vi "Main.vi"() -> ()   [LabVIEW 2017]
doc: "This Continuous Measurement sample project is based on the Queued Message Handler template.\n\nThe Event Handling Loop generates messages based on user interface actions.\n\nThe Message Handling Loop processes messages generated by the Event Handling Loop, or by other messages. There are also Acquisition and Logging message handling loop subVIs, and a chart updating loop."
uses:
  Acquisition/Hardware Configuration.ctl
  Logging/Logging Configuration.ctl
  <vilib>/Analysis/baseanly.llb/Mean (DBL).vi
  <vilib>/express/express analysis/Spectral/Block/exnSpectralBlock spectral measurements PSD poly.vi
  <vilib>/express/express analysis/Spectral/Block/exnSpectralBlock spectral measurements PSD DDT.vi
  support/Message Queue/Enqueue Message (Single).vi
  <vilib>/Utility/error.llb/Error Cluster From Error Code.vi
  <vilib>/express/express analysis/Spectral/XNode/ExpressSpectralMeasurementsBlockNode.xnode
  <vilib>/ErrorRing/Error Ring.xnode
  Acquisition/Acquisition.lvlib
  Logging/Logging.lvlib
  Settings/Settings.lvlib
  support/User Event - Stop/User Event - Stop.lvlib
  support/Message Queue/Message Queue.lvlib
  <vilib>/Analysis/NI_AALBase.lvlib
  <vilib>/gmath/NI_Gmath.lvlib
panel:
  out "XY Graph 4":cluster{"Y":sgl[], "Y":sgl[]}(graph)
  in  "Plot 2":bool
  out "XY Graph 3":cluster{"Y":sgl[], "Y":sgl[]}(graph)
  out "B2Y 2":dbl(graph)=nan
  out "B2X 3":dbl(graph)=nan
  out "B1Y 2":dbl(graph)=nan
  out "B1X 2":dbl(graph)=nan
  out "B2X 2":dbl(graph)
  out "PZTZ0":dbl
  out "PZTY0":dbl
  out "PZTX0":dbl
  in  "PZTZ_offset":dbl caption="Offset" format="%#.0f"
  in  "PZTY_offset":dbl caption="Offset" format="%#.0f"
  in  "PZTX_offset":dbl caption="Offset" format="%#.0f"
  in  "Plot":bool
  in  "PSD":bool
  in  "PZT_offset":bool caption="Offset all"
  out "PZTZ PSD":dynamicdata(graph)=[{"t0"=timestamp(0 s since 1904-01-01), "dt"=inf, "Y"=[], "attributes"=variant("NI_ChannelName"=variant(string "Collected (PSD)"), "NI_OriginalChannelName"=variant(string "Collected"))}]
  out "PZTY PSD":dynamicdata(graph)=[{"t0"=timestamp(0 s since 1904-01-01), "dt"=inf, "Y"=[], "attributes"=variant("NI_ChannelName"=variant(string "Collected (PSD)"), "NI_OriginalChannelName"=variant(string "Collected"))}]
  out "PZTX PSD":dynamicdata(graph)=[{"t0"=timestamp(0 s since 1904-01-01), "dt"=inf, "Y"=[], "attributes"=variant("NI_ChannelName"=variant(string "Collected (PSD)"), "NI_OriginalChannelName"=variant(string "Collected"))}]
  in  "B1X":dbl=1.0
  in  "B1Y":dbl=1.0
  in  "B2X":dbl=1.0
  in  "B2Y":dbl=1.0
  out "Description":string
  out "User":string
  out "Corr":dbl format="%.2g"
  out "XY Graph 2":cluster{"Y":sgl[], "Y":sgl[]}(graph) caption="XY Graph"
  out "Corr":dbl format="%.2g"
  out "XY Graph":cluster{"Y":sgl[], "Y":sgl[]}(graph)
  out "B2S":sgl format="%#_2g"
  out "B2Y":dbl(graph)=nan
  out "B2X":dbl(graph)=nan
  out "B2Y PSD":dynamicdata(graph)=[{"t0"=timestamp(0 s since 1904-01-01), "dt"=inf, "Y"=[], "attributes"=variant("NI_ChannelName"=variant(string "Collected (PSD)"), "NI_OriginalChannelName"=variant(string "Collected"))}]
  out "B2X PSD":dynamicdata(graph)=[{"t0"=timestamp(0 s since 1904-01-01), "dt"=inf, "Y"=[], "attributes"=variant("NI_ChannelName"=variant(string "Collected (PSD)"), "NI_OriginalChannelName"=variant(string "Collected"))}]
  out "B1S":sgl format="%#_2g"
  out "B1Y PSD":dynamicdata(graph)=[{"t0"=timestamp(0 s since 1904-01-01), "dt"=inf, "Y"=[], "attributes"=variant("NI_ChannelName"=variant(string "Collected (PSD)"), "NI_OriginalChannelName"=variant(string "Collected"))}]
  out "B1X PSD":dynamicdata(graph)=[{"t0"=timestamp(0 s since 1904-01-01), "dt"=inf, "Y"=[], "attributes"=variant("NI_ChannelName"=variant(string "Collected (PSD)"), "NI_OriginalChannelName"=variant(string "Collected"))}]
  out "PZTZ":dbl(graph)
  out "PZTY":dbl(graph)
  out "PZTX":dbl(graph)
  out "?":dbl
  out "Input (V)":dbl
  out "Rate (Hz)":dbl
  in  "Stop_Log":bool
  in  "Log":bool
  in  "Exit":bool
  out "Status":string
  in  "Settings":bool
  in  "Stop_Acquire":bool
  in  "Acquire":bool
  out "B1Y":dbl(graph)=nan
  out "B1X":dbl(graph)=nan
  # "nm/V"
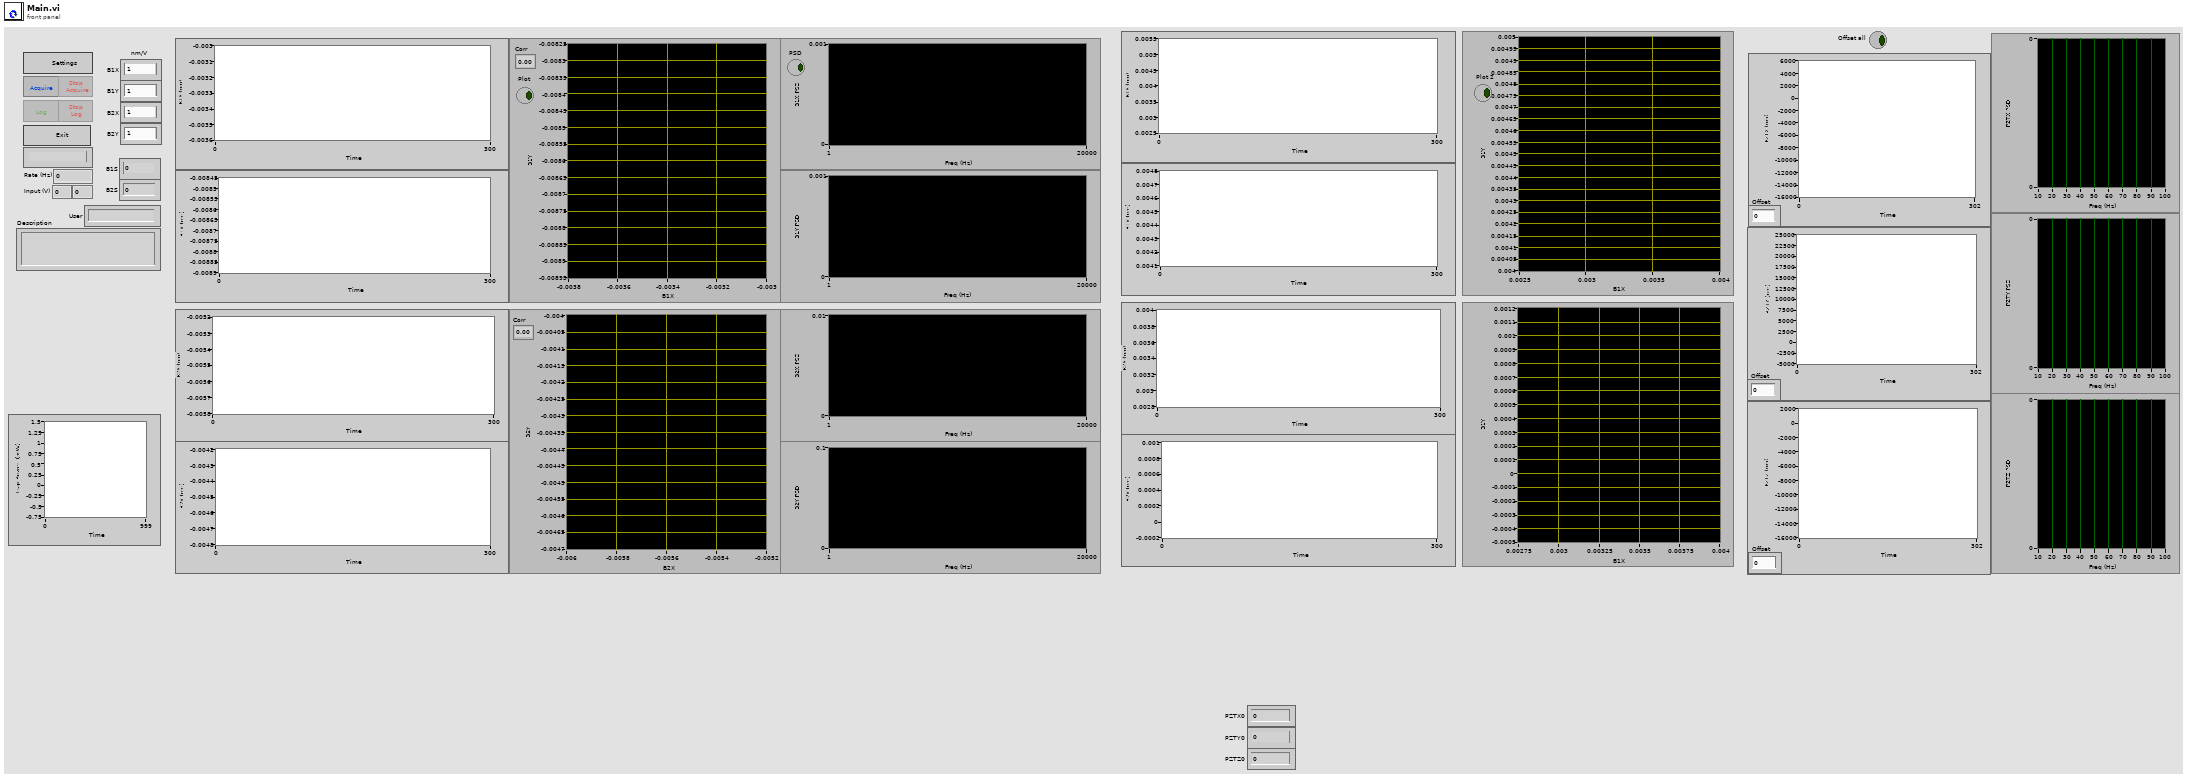
[diagram p1: front panel]
types:
  T1 = cluster{"Acquire Ref":refnum<vi>, "Log Ref":refnum<vi>, "Stop_Acquire Ref":refnum<vi>, "Settings Ref":refnum<vi>, "Status Ref":refnum<vi>, "Exit Ref":refnum<vi>, "Stop_Log Ref":refnum<vi>}
  T2 = typedef "Acquisition.lvlib/Hardware Configuration.ctl" = cluster{"DAQmx Input":tag, "Max Input":dbl, "Min Input":dbl, "Sample Rate":dbl, "DAQmx Task":refnum<k21>}
  T3 = typedef "Logging.lvlib/Logging Configuration.ctl" = cluster{"Log File Base Path":path, "TDMS File Reference":refnum<k34>, "Channel names":string[], "Author":string, "Description":string}
  T4 = cluster{"Hardware Configuration":T2, "Logging Configuration":T3}
  T5 = typedef "Message Queue.lvlib/All Message Queues.ctl" = cluster{"UI":refnum<queue>, "Acquisition":refnum<queue>, "Logging":refnum<queue>}
  T6 = cluster{"averaging mode":u16, "weighting mode":u16, "number of averages":u32}
  T7 = cluster{"dB On (F)":bool, "unwrap phase (F)":bool, "convert to degree (F)":bool}
  T8 = cluster{"Hardware Configuration":T2, "Logging Configuration":cluster{"Log File Base Path":path, "TDMS File Reference":refnum<k34>, "Channel names":string[], "Author":string, "Description":string}}
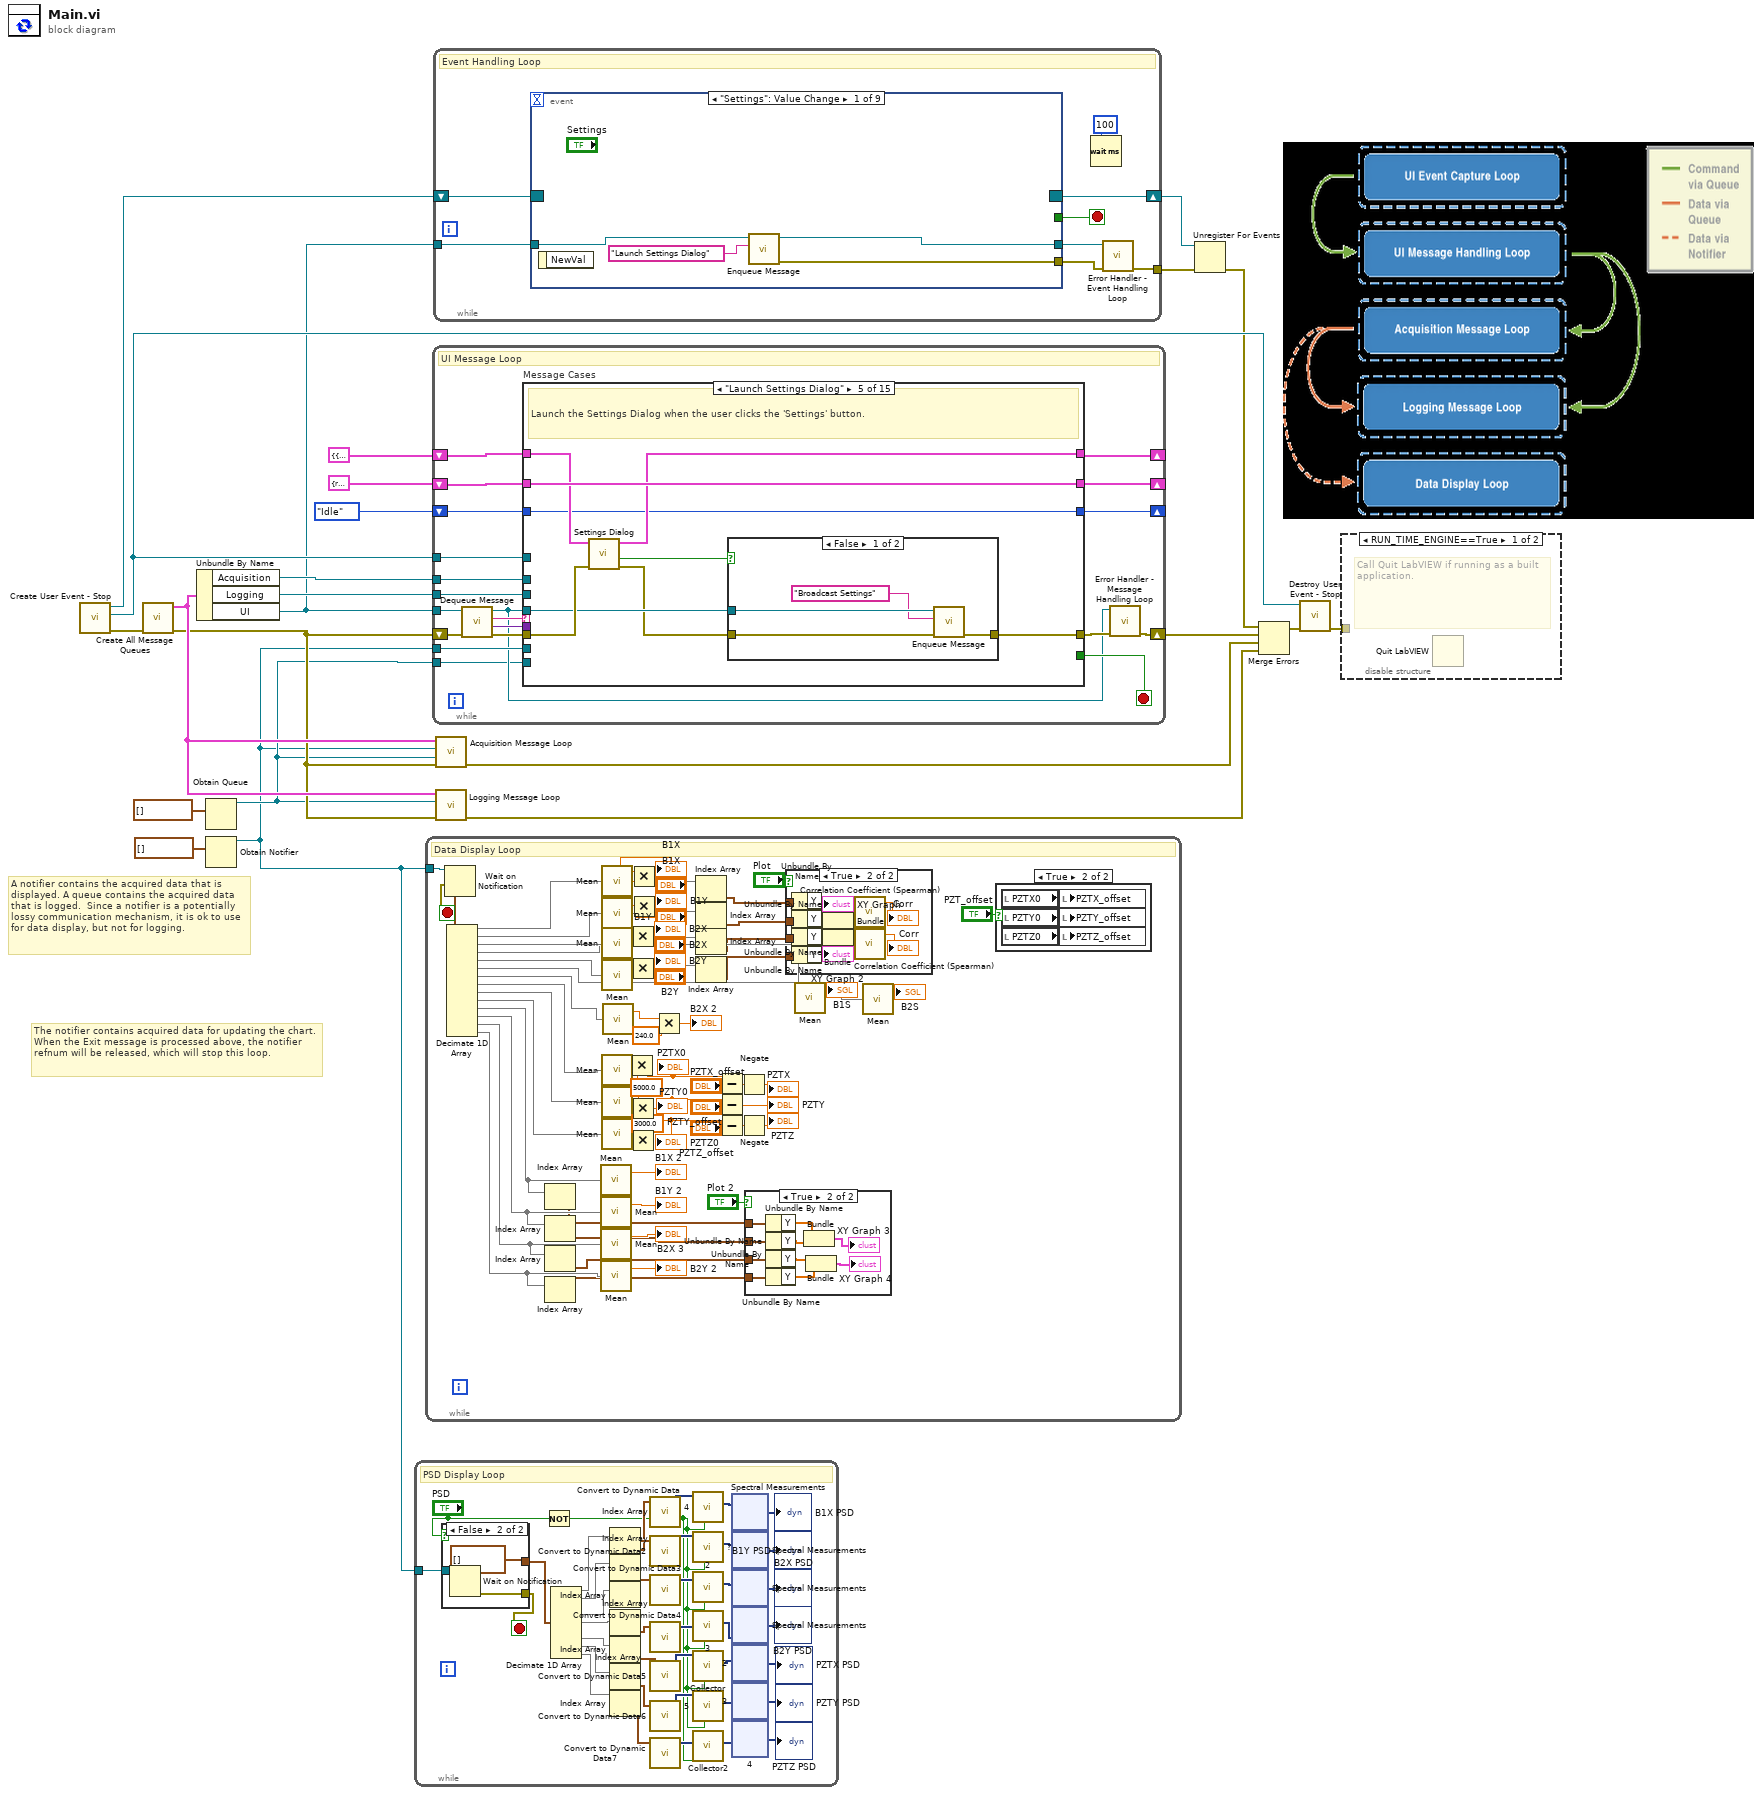
[diagram p0: block diagram]
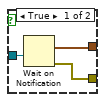
[diagram p2: hidden frame]
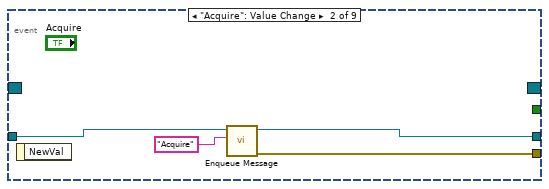
[diagram p7: hidden frame]
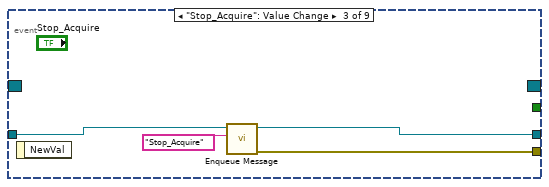
[diagram p8: hidden frame]
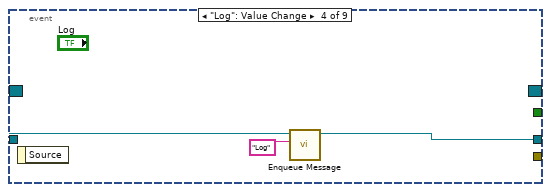
[diagram p9: hidden frame]
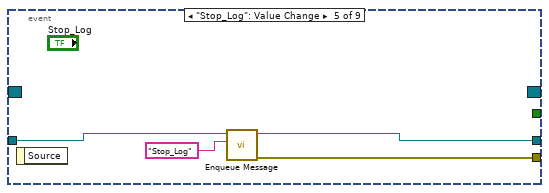
[diagram p10: hidden frame]
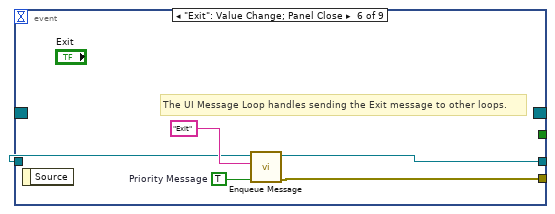
[diagram p11: hidden frame]
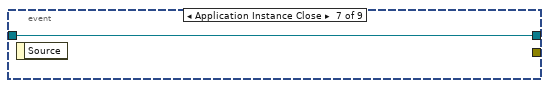
[diagram p12: hidden frame]
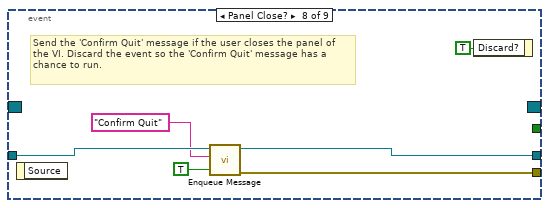
[diagram p13: hidden frame]
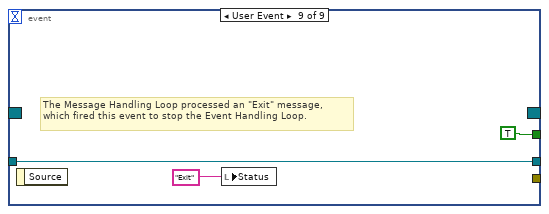
[diagram p14: hidden frame]
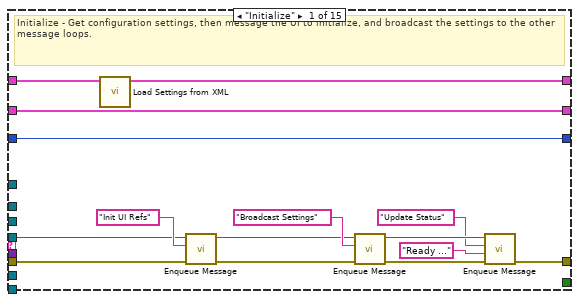
[diagram p15: hidden frame]
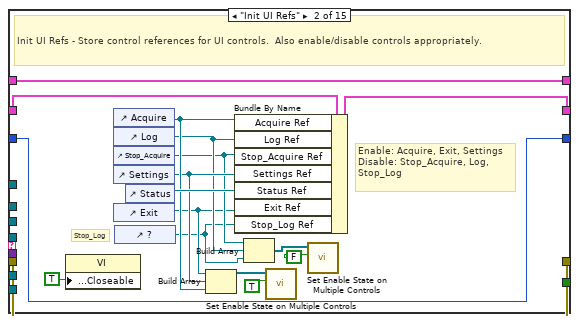
[diagram p16: hidden frame]
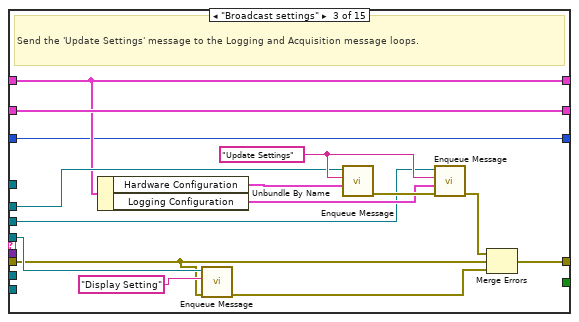
[diagram p17: hidden frame]
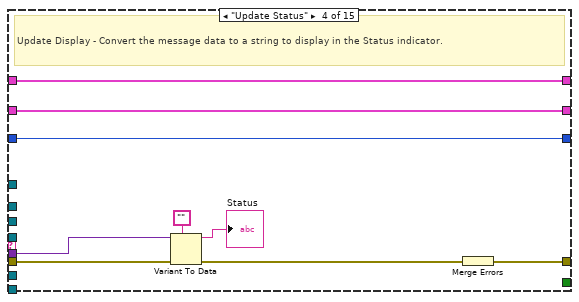
[diagram p18: hidden frame]
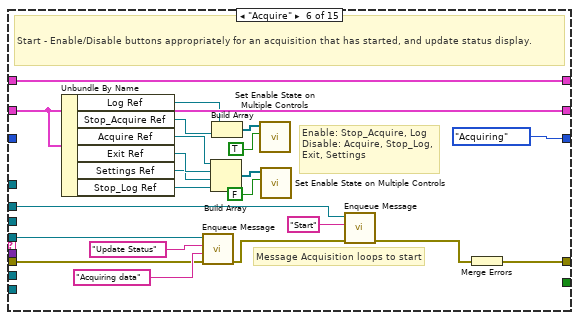
[diagram p20: hidden frame]
diagram:
  # "A notifier contains the acquired data that is displayed. A queue contains the acquired data that is logged.  Since a notifier is a potentially lossy communication mechanism, it is ok to use for data display, but not for logging."
  # "The notifier contains acquired data for updating the chart. When the Exit message is processed above, the notifier refnum will be released, which will stop this loop."
  n1 = call "Create User Event - Stop.vi"() -> ("error out"=w17:errorcluster, "User Event - Stop"=w19:refnum<user-event>, "Stop Event Registration Refnum"=w20:refnum<event-registration>)  [unwired: 9 in]
  n2 = call "Create All Message Queues.vi"("error in (no error)"=w17) -> ("error out"=w4:errorcluster, "Message Queues out"=w16:T5)  [unwired: 9 in]
  n3 = Unbundle By Name(w16) -> ("Acquisition"=w11:refnum<queue>, "Logging"=w10:refnum<queue>, "UI"=w3:refnum<queue>)
  n4 = Obtain Queue(element data type=waveform(sgl)[] []) -> (queue out=w2:refnum<queue>)  [unwired: 4 in, 2 out]
  n5 = Obtain Notifier(notification data type=waveform(sgl)[] []) -> (notifier out=w1:refnum<notifier>)  [unwired: 3 in, 2 out]
  n6 = while {
    tunnel: w1 -> [w62]
    stop <- w24 stop-if-true
    # "PSD Display Loop"
    n7 = case shown="False" "PSD" {
      tunnel: [w66 waveform(sgl)[] []] -> w63
      tunnel: w62 -> [w65 w69]
      tunnel: [w64 w68] -> w24
      frame True {
        n8 = Wait on Notification(notifier=w65) -> (notification=w66:waveform(sgl)[], error out=w64:errorcluster)  [unwired: 3 in, 2 out]
      }
      frame False {
        n9 = Wait on Notification(notifier=w69) -> (error out=w68:errorcluster)  [unwired: 3 in, 3 out]
      }
    }
    n10 = Not(x="PSD") -> (.not. x?=w33:bool)
    n11 = Decimate 1D Array(w63) -> (w53:waveform(sgl)[], w52:waveform(sgl)[], w51:waveform(sgl)[], w50:waveform(sgl)[], w42:waveform(sgl)[], w41:waveform(sgl)[], w40:waveform(sgl)[])  [unwired: 2 out]
    n12 = Index Array(array=w53) -> (element=w58:waveform(sgl))  [unwired: 1 in]
    n13 = Index Array(array=w52) -> (element=w59:waveform(sgl))  [unwired: 1 in]
    n14 = Index Array(array=w51) -> (element=w60:waveform(sgl))  [unwired: 1 in]
    n15 = Index Array(array=w50) -> (element=w61:waveform(sgl))  [unwired: 1 in]
    n16 = Index Array(array=w42) -> (element=w45:waveform(sgl))  [unwired: 1 in]
    n17 = Index Array(array=w41) -> (element=w44:waveform(sgl))  [unwired: 1 in]
    n18 = Index Array(array=w40) -> (element=w43:waveform(sgl))  [unwired: 1 in]
    n19 = call "Convert to Dynamic Data"("Waveform"=w58) -> ("Dynamic Data Type"=w57:dynamicdata)  [unwired: 3 in]
    n20 = call "Convert to Dynamic Data2"("Waveform"=w59) -> ("Dynamic Data Type"=w54:dynamicdata)  [unwired: 3 in]
    n21 = call "Convert to Dynamic Data3"("Waveform"=w60) -> ("Dynamic Data Type"=w55:dynamicdata)  [unwired: 3 in]
    n22 = call "Convert to Dynamic Data4"("Waveform"=w61) -> ("Dynamic Data Type"=w56:dynamicdata)  [unwired: 3 in]
    n23 = call "Convert to Dynamic Data5"("Waveform"=w45) -> ("Dynamic Data Type"=w39:dynamicdata)  [unwired: 3 in]
    n24 = call "Convert to Dynamic Data6"("Waveform"=w44) -> ("Dynamic Data Type"=w37:dynamicdata)  [unwired: 3 in]
    n25 = call "Convert to Dynamic Data7"("Waveform"=w43) -> ("Dynamic Data Type"=w36:dynamicdata)  [unwired: 3 in]
    n26 = call "4"("Reset"=w33, "Signals"=w57) -> ("Collected Signals"=w49:dynamicdata)  [unwired: 8 in, 1 out]
    n27 = call "?"("Reset"=w33, "Signals"=w54) -> ("Collected Signals"=w48:dynamicdata)  [unwired: 8 in, 1 out]
    n28 = call "2"("Reset"=w33, "Signals"=w55) -> ("Collected Signals"=w47:dynamicdata)  [unwired: 8 in, 1 out]
    n29 = call "3"("Reset"=w33, "Signals"=w56) -> ("Collected Signals"=w46:dynamicdata)  [unwired: 8 in, 1 out]
    n30 = call "Collector"("Reset"=w33, "Signals"=w39) -> ("Collected Signals"=w38:dynamicdata)  [unwired: 8 in, 1 out]
    n31 = call "5"("Reset"=w33, "Signals"=w37) -> ("Collected Signals"=w35:dynamicdata)  [unwired: 8 in, 1 out]
    n32 = call "Collector2"("Reset"=w33, "Signals"=w36) -> ("Collected Signals"=w34:dynamicdata)  [unwired: 8 in, 1 out]
    n33 = xnode ("Spectral Measurements")("Signals"=w49) -> ("PSD"=→"B1X PSD":dynamicdata)  [unwired: 2 in, 2 out]
    n34 = xnode ("Spectral Measurements")("Signals"=w48) -> ("PSD"=→"B1Y PSD":dynamicdata)  [unwired: 2 in, 2 out]
    n35 = xnode ("Spectral Measurements")("Signals"=w47) -> ("PSD"=→"B2X PSD":dynamicdata)  [unwired: 2 in, 2 out]
    n36 = xnode ("Spectral Measurements")("Signals"=w46) -> ("PSD"=→"B2Y PSD":dynamicdata)  [unwired: 2 in, 2 out]
    n37 = xnode ("2")("Signals"=w38) -> ("PSD"=→"PZTX PSD":dynamicdata)  [unwired: 2 in, 2 out]
    n38 = xnode ("3")("Signals"=w35) -> ("PSD"=→"PZTY PSD":dynamicdata)  [unwired: 2 in, 2 out]
    n39 = xnode ("4")("Signals"=w34) -> ("PSD"=→"PZTZ PSD":dynamicdata)  [unwired: 2 in, 2 out]
  }
  n40 = while "Data Display Loop" {
    tunnel: w1 -> [w204]
    stop <- w174 stop-if-true
    w175 = 5000.0 ("y")
    # "Data Display Loop"
    n41 = Wait on Notification(notifier=w204) -> (notification=w203:waveform(sgl)[], error out=w174:errorcluster)  [unwired: 3 in, 2 out]
    n42 = Decimate 1D Array(w203) -> (w183:waveform(sgl)[], w181:waveform(sgl)[], w201:waveform(sgl)[], w178:waveform(sgl)[], w176:waveform(sgl)[], w200:waveform(sgl)[], w152:waveform(sgl)[], w151:waveform(sgl)[], w150:waveform(sgl)[], w149:waveform(sgl)[], w148:waveform(sgl)[], w147:waveform(sgl)[], w146:waveform(sgl)[], w145:waveform(sgl)[])
    n43 = Index Array(array=w148) -> (element=w144:waveform(sgl))  [unwired: 1 in]
    n44 = Index Array(array=w147) -> (element=w143:waveform(sgl))  [unwired: 1 in]
    n45 = Index Array(array=w146) -> (element=w142:waveform(sgl))  [unwired: 1 in]
    n46 = Index Array(array=w145) -> (element=w141:waveform(sgl))  [unwired: 1 in]
    n47 = call-poly <vilib>:"Mean.vi"("X"=w148) -> ("mean"=→"B1X 2":dbl)  [unwired: 1 out]
    n48 = call-poly <vilib>:"Mean.vi"("X"=w147) -> ("mean"=→"B1Y 2":dbl)  [unwired: 1 out]
    n49 = call-poly <vilib>:"Mean.vi"("X"=w146) -> ("mean"=→"B2X 3":dbl)  [unwired: 1 out]
    n50 = call-poly <vilib>:"Mean.vi"("X"=w145) -> ("mean"=→"B2Y 2":dbl)  [unwired: 1 out]
    n51 = call-poly <vilib>:"Mean.vi"("X"=w183) -> ("mean"=w182:dbl)  [unwired: 1 out]
    n52 = call-poly <vilib>:"Mean.vi"("X"=w181) -> ("mean"=w180:dbl)  [unwired: 1 out]
    n53 = call-poly <vilib>:"Mean.vi"("X"=w178) -> ("mean"=w179:dbl)  [unwired: 1 out]
    n54 = call-poly <vilib>:"Mean.vi"("X"=w176) -> ("mean"=w177:dbl)  [unwired: 1 out]
    n55 = call-poly <vilib>:"Mean.vi"("X"=w151) -> ("mean"=w170:dbl)  [unwired: 1 out]
    n56 = call-poly <vilib>:"Mean.vi"("X"=w150) -> ("mean"=w169:dbl)  [unwired: 1 out]
    n57 = call-poly <vilib>:"Mean.vi"("X"=w149) -> ("mean"=w168:dbl)  [unwired: 1 out]
    n58 = call-poly <vilib>:"Mean.vi"("X"=w152) -> ("mean"=w161:dbl)  [unwired: 1 out]
    n59 = Multiply(x=w170, y=w175) -> (x*y=w173:dbl)
    "PZTX0" <- w173
    n60 = Multiply(x=w179, y="B2X") -> (x*y=→"B2X":dbl)
    n61 = Multiply(x=w177, y="B2Y") -> (x*y=→"B2Y":dbl)
    n62 = Multiply(x=w169, y=w175) -> (x*y=w193:dbl)
    "PZTY0" <- w193
    n63 = Multiply(x=w168, y=3000.0) -> (x*y=w165:dbl)
    "PZTZ0" <- w165
    n64 = Multiply(x=w182, y="B1X") -> (x*y=→"B1X":dbl)
    n65 = Multiply(x=w180, y="B1Y") -> (x*y=→"B1Y":dbl)
    n66 = Multiply(x=w161, y=240.0) -> (x*y=→"B2X 2":dbl)
    n67 = Index Array(array=w183) -> (element=w197:waveform(sgl))  [unwired: 1 in]
    n68 = Index Array(array=w181) -> (element=w196:waveform(sgl))  [unwired: 1 in]
    n69 = Index Array(array=w178) -> (element=w195:waveform(sgl))  [unwired: 1 in]
    n70 = Index Array(array=w176) -> (element=w194:waveform(sgl))  [unwired: 1 in]
    n71 = Subtract(x=w173, y="PZTX_offset") -> (x-y=w172:dbl)
    n72 = Subtract(x=w193, y="PZTY_offset") -> (x-y=→"PZTY":dbl)
    n73 = Subtract(x=w165, y="PZTZ_offset") -> (x-y=w171:dbl)
    n74 = Negate(x=w172) -> (-x=→"PZTX":dbl)
    n75 = Negate(x=w171) -> (-x=→"PZTZ":dbl)
    n76 = case shown="True" "Plot 2" {
      tunnel: w144 -> [_ w209]
      tunnel: w143 -> [_ w208]
      tunnel: w142 -> [_ w206]
      tunnel: w141 -> [_ w207]
      frame False {
      }
      frame True {
        n77 = Unbundle By Name(w209) -> ("Y"=w214:sgl[])
        n78 = Unbundle By Name(w208) -> ("Y"=w213:sgl[])
        n79 = Unbundle By Name(w206) -> ("Y"=w212:sgl[])
        n80 = Unbundle By Name(w207) -> ("Y"=w211:sgl[])
        n81 = Bundle("Y"=w214, "Y"=w213) -> (→"XY Graph 3":cluster{"Y":sgl[], "Y":sgl[]})  [unwired: 1 in]
        n82 = Bundle("Y"=w212, "Y"=w211) -> (→"XY Graph 4":cluster{"Y":sgl[], "Y":sgl[]})  [unwired: 1 in]
      }
    }
    n83 = case shown="True" "Plot" {
      tunnel: w197 -> [_ w221]
      tunnel: w196 -> [_ w220]
      tunnel: w195 -> [_ w219]
      tunnel: w194 -> [_ w218]
      frame False {
      }
      frame True {
        n84 = Unbundle By Name(w221) -> ("Y"=w227:sgl[])
        n85 = Unbundle By Name(w220) -> ("Y"=w226:sgl[])
        n86 = Unbundle By Name(w219) -> ("Y"=w223:sgl[])
        n87 = Unbundle By Name(w218) -> ("Y"=w222:sgl[])
        n88 = Bundle("Y"=w227, "Y"=w226) -> (→"XY Graph":cluster{"Y":sgl[], "Y":sgl[]})  [unwired: 1 in]
        n89 = Bundle("Y"=w223, "Y"=w222) -> (→"XY Graph 2":cluster{"Y":sgl[], "Y":sgl[]})  [unwired: 1 in]
        n90 = call <vilib>:"Correlation Coefficient (Spearman).vi"("Y"=w226, "X"=w227) -> ("correlation coefficient r"=→"Corr":dbl)  [unwired: 8 in, 1 out]
        n91 = call <vilib>:"Correlation Coefficient (Spearman).vi"("Y"=w222, "X"=w223) -> ("correlation coefficient r"=→"Corr":dbl)  [unwired: 8 in, 1 out]
      }
    }
    n92 = call-poly <vilib>:"Mean.vi"("X"=w201) -> ("mean"=→"B1S":dbl)  [unwired: 1 out]
    n93 = call-poly <vilib>:"Mean.vi"("X"=w200) -> ("mean"=→"B2S":dbl)  [unwired: 1 out]
    n94 = case shown="True" "PZT_offset" {
      frame False {
      }
      frame True {
        n95 = local read "PZTX0"() -> (w217:dbl)
        n96 = local read "PZTY0"() -> (w216:dbl)
        n97 = local read "PZTZ0"() -> (w215:dbl)
        n98 = local write "PZTX_offset"(w217) -> ()
        n99 = local write "PZTY_offset"(w216) -> ()
        n100 = local write "PZTZ_offset"(w215) -> ()
      }
    }
  }
  n101 = while {
    tunnel: w3 -> [w243]
    tunnel: w19 -> [w248]
    shift-right: [w236] -> w23
    shift-left: w4 -> [w247]
    shift-right: [w234] -> _
    shift-left: T4 {"Hardware Configuration"={"DAQmx Input"="", "Max Input"=0.0, "Min Input"=0.0, "Sample Rate"=0.0, "DAQmx Task"=""}, "Logging Configuration"={"Log File Base Path"=path "", "TDMS File Reference"=refnum, "Channel names"=[], "Author"="", "Description"=""}} ("Settings") -> [w230]
    shift-right: [w241] -> _
    shift-left: T1 {"Acquire Ref"=refnum, "Log Ref"=refnum, "Stop_Acquire Ref"=refnum, "Settings Ref"=refnum, "Status Ref"=refnum, "Exit Ref"=refnum, "Stop_Log Ref"=refnum} ("Measurement UI Controls") -> [w242]
    tunnel: w11 -> [w240]
    tunnel: w10 -> [w239]
    tunnel: w1 -> [w238]
    shift-right: [w233] -> _
    shift-left: enum16{"Idle", "Acquiring", "Logging"}."Idle" ("UI State") -> [w232]
    tunnel: w2 -> [w231]
    stop <- w249 stop-if-true
    # "UI Message Loop"
    n102 = call "Dequeue Message.vi"("error in (no error)"=w247, "Message Queue"=w243) -> ("error out"=w246:errorcluster, "Message Data"=w244:variant, "Message"=w245:string, "dup Message Queue"=w235:refnum<queue>)  [unwired: 6 in]
    n103 = case "Message Cases" shown="\"Launch Settings Dialog\"" w245 {
      selector: w245 -> [_ _ _ _ _ _ _ _ _ _ _ _ _ _ w499]
      tunnel: w235 -> [w256 _ w287 _ w312 w340 w345 w385 w391 w420 w438 w476 _ _ _]
      tunnel: w246 -> [w255 w281 w285 w304 w314 w322 w347 w387 w410 w427 w435 w480 w486 w496 _]
      tunnel: [w262 w281 w296 w305 w310 w341 w364 w386 w409 w428 w434 w471 w485 w495 w500] -> w237
      tunnel: [_ _ _ _ _ _ _ _ _ TRUE _ _ _ _ _] -> w249
      tunnel: w244 -> [_ _ _ w303 _ _ _ _ _ _ _ w479 _ _ _]
      tunnel: w248 -> [_ _ _ _ _ _ _ _ _ w426 _ _ _ _ _]
      tunnel: w230 -> [w252 w266 w283 w298 w308 w321 w349 w369 w395 w413 w432 w470 w483 w490 w498]
      tunnel: w242 -> [w258 w280 w290 w300 w309 w337 w363 w382 w408 w423 w439 w481 w484 w494 w501]
      tunnel: [w258 w279 w290 w300 w309 w337 w363 w382 w408 w423 w439 w481 w484 w494 w501] -> w241
      tunnel: w240 -> [_ _ w289 _ _ w328 w359 w367 w393 w422 w437 _ _ _ _]
      tunnel: w239 -> [_ _ w288 _ _ _ _ w379 w405 w421 w436 _ _ _ _]
      tunnel: w238 -> [_ _ _ _ _ _ _ _ _ w419 _ _ _ _ _]
      tunnel: [w251 w266 w283 w298 w307 w321 w349 w369 w395 w413 w432 w470 w483 w490 w498] -> w234
      tunnel: [w250 w265 w282 w297 w306 enum16{"Idle", "Acquiring", "Logging"}."Acquiring" ("UI State") enum16{"Idle", "Acquiring", "Logging"}."Idle" ("UI State") enum16{"Idle", "Acquiring", "Logging"}."Logging" ("UI State") enum16{"Idle", "Acquiring", "Logging"}."Acquiring" ("UI State") enum16{"Idle", "Acquiring", "Logging"}."Idle" ("UI State") w431 w469 w482 w487 w497] -> w233
      tunnel: w232 -> [w250 w265 w282 w297 w306 _ _ _ _ _ w430 w469 w482 w487 w497]
      tunnel: w231 -> [_ _ _ _ _ _ _ _ _ w411 _ _ _ _ _]
      frame "Initialize" {
        # "Initialize - Get configuration settings, then message the UI to initialize, and broadcast the settings to the other message loops."
        n104 = call "Load Settings from XML.vi"("Settings in"=w252) -> ("Settings out"=w251:T4)  [unwired: 9 in, 1 out]
        n105 = call-poly "Enqueue Message.vi"("error in (no error)"=w255, "Message"="Init UI Refs", "Message Queue"=w256) -> ("error out"=w253:errorcluster, "dup Message Queue"=w254:refnum<queue>)  [unwired: 7 in]
        n106 = call-poly "Enqueue Message.vi"("error in (no error)"=w253, "Message"="Broadcast Settings", "Message Queue"=w254) -> ("error out"=w264:errorcluster, "dup Message Queue"=w263:refnum<queue>)  [unwired: 7 in]
        n107 = call-poly "Enqueue Message.vi"("error in (no error)"=w264, "Message Data"="Ready ..." ("Ready..."), "Message"="Update Status", "Message Queue"=w263) -> ("error out"=w262:errorcluster)  [unwired: 6 in, 1 out]
      }
      frame "Init UI Refs" {
        # "Stop_Log"
        # "Enable: Acquire, Exit, Settings\nDisable: Stop_Acquire, Log, Stop_Log"
        # "Init UI Refs - Store control references for UI controls.  Also enable/disable controls appropriately."
        n108 = property class="VI"("Front Panel.Closeable"=TRUE ("Front Panel Window:Closeable")) -> ()  [unwired: 2 in, 2 out]
        n109 = control-ref of="Acquire"() -> (w275:refnum<vi>)
        n110 = control-ref of="Log"() -> (w271:refnum<vi>)
        n111 = control-ref of="Stop_Acquire"() -> (w270:refnum<vi>)
        n112 = control-ref of="Settings"() -> (w272:refnum<vi>)
        n113 = control-ref of="Exit"() -> (w268:refnum<vi>)
        n114 = control-ref of="?"() -> (w267:refnum<vi>)
        n115 = control-ref of="Status"() -> (w276:refnum<vi>)
        n116 = Build Array(w268, w272, w275) -> (w274:refnum<vi>[])
        n117 = Bundle By Name(cluster=w280, "Acquire Ref"=w275, "Log Ref"=w271, "Stop_Acquire Ref"=w270, "Settings Ref"=w272, "Status Ref"=w276, "Exit Ref"=w268, "Stop_Log Ref"=w267) -> (w279:T1)
        n118 = Build Array(w270, w271, w267) -> (w269:refnum<vi>[])
        n119 = call "Set Enable State on Multiple Controls.vi"("Enable?"=TRUE, "Controls"=w274) -> ()  [unwired: 10 in]
        n120 = call "Set Enable State on Multiple Controls.vi"("Enable?"=FALSE, "Controls"=w269) -> ()  [unwired: 10 in]
      }
      frame "Broadcast settings" {
        w291 = "Update Settings" ("Message")
        # "Send the 'Update Settings' message to the Logging and Acquisition message loops."
        n121 = Unbundle By Name(w283) -> ("Hardware Configuration"=w294:T2, "Logging Configuration"=w293:T3)
        n122 = call-poly "Enqueue Message.vi"("error in (no error)"=w285, "Message"="Display Setting", "Message Queue"=w287) -> ("error out"=w284:errorcluster)  [unwired: 7 in, 1 out]
        n123 = call-poly "Enqueue Message.vi"("Message Data"=w294, "Message"=w291, "Message Queue"=w289) -> ("error out"=w295:errorcluster)  [unwired: 7 in, 1 out]
        n124 = call-poly "Enqueue Message.vi"("error in (no error)"=w295, "Message Data"=w293, "Message"=w291, "Message Queue"=w288) -> ("error out"=w292:errorcluster)  [unwired: 6 in, 1 out]
        n125 = Merge Errors(w292, w285, w284) -> (w296:errorcluster)
      }
      frame "Update Status" {
        # "Update Display - Convert the message data to a string to display in the Status indicator."
        n126 = Variant To Data(error in=w304, type="", Variant=w303) -> (data=→"Status":string, error out=w301:errorcluster)
        n127 = Merge Errors(w301) -> (w305:errorcluster)
      }
      frame "Launch Settings Dialog" {
        # "Launch the Settings Dialog when the user clicks the 'Settings' button."
        n128 = call "Settings Dialog.vi"("error in (no error)"=w314, "Settings in"=w308) -> ("error out"=w311:errorcluster, "Cancelled?"=w313:bool, "Settings out"=w307:T8)  [unwired: 6 in, 1 out]
        n129 = case shown="False" w313 {
          tunnel: w312 -> [w318 _]
          tunnel: w311 -> [w317 w319]
          tunnel: [w316 w319] -> w310
          frame False {
            n130 = call-poly "Enqueue Message.vi"("error in (no error)"=w317, "Message"="Broadcast Settings", "Message Queue"=w318) -> ("error out"=w316:errorcluster)  [unwired: 7 in, 1 out]
          }
          frame True {
          }
        }
      }
      frame "Acquire" {
        # "Message Acquisition loops to start"
        # "Enable: Stop_Acquire, Log\nDisable: Acquire, Stop_Log, Exit, Settings"
        # "Start - Enable/Disable buttons appropriately for an acquisition that has started, and update status display."
        n131 = Unbundle By Name(w337) -> ("Log Ref"=w325:refnum<vi>, "Stop_Acquire Ref"=w326:refnum<vi>, "Acquire Ref"=w332:refnum<vi>, "Exit Ref"=w331:refnum<vi>, "Settings Ref"=w330:refnum<vi>, "Stop_Log Ref"=w323:refnum<vi>)
        n132 = call-poly "Enqueue Message.vi"("error in (no error)"=w322, "Message Data"="Acquiring data" ("Waiting for trigger"), "Message"="Update Status", "Message Queue"=w340) -> ("error out"=w324:errorcluster)  [unwired: 6 in, 1 out]
        n133 = Build Array(w332, w331, w330, w323) -> (w335:refnum<vi>[])
        n134 = Build Array(w325, w326) -> (w334:refnum<vi>[])
        n135 = call "Set Enable State on Multiple Controls.vi"("Enable?"=TRUE, "Controls"=w334) -> ()  [unwired: 10 in]
        n136 = call "Set Enable State on Multiple Controls.vi"("Enable?"=FALSE, "Controls"=w335) -> ()  [unwired: 10 in]
        n137 = call-poly "Enqueue Message.vi"("error in (no error)"=w324, "Message"="Start", "Message Queue"=w328) -> ("error out"=w329:errorcluster)  [unwired: 7 in, 1 out]
        n138 = Merge Errors(w329) -> (w341:errorcluster)
      }
      frame "Stop_Acquire" {
        # "Message Acquisition loop to stop"
        # "Enable: Acquire, Exit, Settings\nDisable: Stop_Acquire, Log, Stop_Log"
        # "Stop - Enable/Disable buttons appropriately for an acquisition that has stopped, and update status display."
        n139 = Unbundle By Name(w363) -> ("Log Ref"=w357:refnum<vi>, "Stop_Acquire Ref"=w356:refnum<vi>, "Acquire Ref"=w355:refnum<vi>, "Exit Ref"=w354:refnum<vi>, "Settings Ref"=w353:refnum<vi>, "Stop_Log Ref"=w352:refnum<vi>)
        n140 = call-poly "Enqueue Message.vi"("error in (no error)"=w347, "Message Data"="Ready..." ("Message"), "Message"="Update Status", "Message Queue"=w345) -> ("error out"=w346:errorcluster)  [unwired: 6 in, 1 out]
        n141 = Build Array(w357, w356, w352) -> (w350:refnum<vi>[])
        n142 = Build Array(w355, w354, w353) -> (w351:refnum<vi>[])
        n143 = call "Set Enable State on Multiple Controls.vi"("Enable?"=TRUE, "Controls"=w351) -> ()  [unwired: 10 in]
        n144 = call "Set Enable State on Multiple Controls.vi"("Enable?"=FALSE, "Controls"=w350) -> ()  [unwired: 10 in]
        n145 = call-poly "Enqueue Message.vi"("Priority Message? (F)"=TRUE, "error in (no error)"=w346, "Message"="Stop", "Message Queue"=w359) -> ("error out"=w360:errorcluster)  [unwired: 6 in, 1 out]
        n146 = Merge Errors(w360) -> (w364:errorcluster)
      }
      frame "Log" {
        # "Enable: Stop_Log\nDisable: Acquire, Stop_Acquire, Exit, Settings, Log"
        # "Duplicate this frame when creating new messages.  Change this comment in the duplicated frame to describe this message."
        n147 = Flush Queue(queue=w367) -> (queue out=w366:refnum<queue>)  [unwired: 1 in, 2 out]
        n148 = call-poly "Enqueue Message.vi"("Message"="Acquire_Log", "Message Queue"=w366) -> ()  [unwired: 8 in, 2 out]
        n149 = Unbundle By Name(w382) -> ("Stop_Log Ref"=w377:refnum<vi>, "Stop_Acquire Ref"=w375:refnum<vi>, "Acquire Ref"=w374:refnum<vi>, "Exit Ref"=w373:refnum<vi>, "Settings Ref"=w372:refnum<vi>, "Log Ref"=w371:refnum<vi>)
        n150 = call-poly "Enqueue Message.vi"("Message Data"="Logging data" ("Ready..."), "Message"="Update Status", "Message Queue"=w385) -> ()  [unwired: 7 in, 2 out]
        n151 = Build Array(w377) -> (w376:refnum<vi>[])
        n152 = Build Array(w375, w374, w373, w372, w371) -> (w370:refnum<vi>[])
        n153 = call "Set Enable State on Multiple Controls.vi"("Enable?"=TRUE, "Controls"=w376) -> ()  [unwired: 10 in]
        n154 = call-poly "Enqueue Message.vi"("Message"="Start", "Message Queue"=w379) -> ()  [unwired: 8 in, 2 out]
        n155 = call "Set Enable State on Multiple Controls.vi"("Enable?"=FALSE, "Controls"=w370) -> ()  [unwired: 10 in]
        n156 = Merge Errors(w387) -> (w386:errorcluster)
      }
      frame "Stop_Log" {
        # "Message Logging loop to stop"
        # "Enable: Log, Stop_Acquire\nDisable: Acquire, Exit, Settings, Stop_Log"
        # "Duplicate this frame when creating new messages.  Change this comment in the duplicated frame to describe this message."
        n157 = Flush Queue(queue=w393) -> (queue out=w392:refnum<queue>)  [unwired: 1 in, 2 out]
        n158 = call-poly "Enqueue Message.vi"("Message"="Acquire", "Message Queue"=w392) -> ()  [unwired: 8 in, 2 out]
        n159 = call-poly "Enqueue Message.vi"("Message"="Stop", "Message Queue"=w405) -> ()  [unwired: 8 in, 2 out]
        n160 = call-poly "Enqueue Message.vi"("Message Data"="Acquiring data" ("Ready..."), "Message"="Update Status", "Message Queue"=w391) -> ()  [unwired: 7 in, 2 out]
        n161 = Unbundle By Name(w408) -> ("Stop_Acquire Ref"=w403:refnum<vi>, "Log Ref"=w397:refnum<vi>, "Acquire Ref"=w401:refnum<vi>, "Exit Ref"=w400:refnum<vi>, "Settings Ref"=w399:refnum<vi>, "Stop_Log Ref"=w396:refnum<vi>)
        n162 = Build Array(w403, w397) -> (w402:refnum<vi>[])
        n163 = Build Array(w396, w401, w400, w399) -> (w398:refnum<vi>[])
        n164 = call "Set Enable State on Multiple Controls.vi"("Enable?"=TRUE, "Controls"=w402) -> ()  [unwired: 10 in]
        n165 = call "Set Enable State on Multiple Controls.vi"("Enable?"=FALSE, "Controls"=w398) -> ()  [unwired: 10 in]
        n166 = Merge Errors(w410) -> (w409:errorcluster)
      }
      frame "Exit" {
        w424 = "Exit" ("Message")
        # "Stop the VI"
        # "Exit - Fire the User Event to stop the Event Handling Loop.  Also send Exit messages to the Acquisition and Logging loops."
        n167 = Release Queue(queue=w420, error in (no error)=w427) -> (error out=w418:errorcluster)  [unwired: 1 in, 2 out]
        n168 = call "Fire User Event - Stop.vi"("User Event - Stop"=w426) -> ("error out"=w425:errorcluster)  [unwired: 10 in]
        n169 = Release Notifier(notifier=w419, error in (no error)=w418) -> (error out=w417:errorcluster)  [unwired: 1 in, 2 out]
        n170 = call-poly "Enqueue Message.vi"("Priority Message? (F)"=TRUE, "Message"=w424, "Message Queue"=w422) -> ()  [unwired: 7 in, 2 out]
        n171 = Release Queue(queue=w411, error in (no error)=w417) -> (error out=w416:errorcluster)  [unwired: 1 in, 2 out]
        n172 = call-poly "Enqueue Message.vi"("Priority Message? (F)"=TRUE, "Message"=w424, "Message Queue"=w421) -> ()  [unwired: 7 in, 2 out]
        n173 = Merge Errors(w425, w416) -> (w428:errorcluster)
      }
      frame "Confirm Quit" {
        # "Confirm Quit - Message that can confirm whether or not the user wants to exit the application."
        n174 = while {
          tunnel: w438 -> [w448]
          tunnel: w437 -> [w447]
          tunnel: w436 -> [w446]
          shift-right: [w442] -> w433
          shift-left: w435 -> [w445]
          shift-right: [w444] -> w431
          shift-left: w430 -> [w443]
          stop <- w441 stop-if-true
          n175 = case shown="\"Logging\"" w443 {
            selector: w443 -> [w450 _ _]
            tunnel: [w452 w455 w463] -> w442
            tunnel: [w450 enum16{"Idle", "Acquiring", "Logging"}."Idle" ("UI State") enum16{"Idle", "Acquiring", "Logging"}."Acquiring" ("UI State")] -> w444
            tunnel: w448 -> [w451 _ _]
            tunnel: w447 -> [_ w459 _]
            tunnel: w445 -> [_ w456 w462]
            tunnel: w446 -> [_ _ w468]
            tunnel: [TRUE ("Priority Message? (F)") FALSE ("Priority Message? (F)") FALSE ("Priority Message? (F)")] -> w441
            frame "Idle", Default {
              n176 = call-poly "Enqueue Message.vi"("Priority Message? (F)"=TRUE, "Message"="Exit", "Message Queue"=w451) -> ("error out"=w452:errorcluster)  [unwired: 7 in, 1 out]
            }
            frame "Acquiring" {
              n177 = call-poly "Enqueue Message.vi"("Priority Message? (F)"=TRUE, "error in (no error)"=w456, "Message"="Stop", "Message Queue"=w459) -> ("error out"=w455:errorcluster)  [unwired: 6 in, 1 out]
            }
            frame "Logging" {
              n178 = call-poly "Enqueue Message.vi"("Priority Message? (F)"=TRUE, "error in (no error)"=w462, "Message"="Stop", "Message Queue"=w468) -> ("error out"=w463:errorcluster)  [unwired: 6 in, 1 out]
            }
          }
          n179 = Wait (ms)(milliseconds to wait=u32 100) -> ()  [unwired: 1 out]
        }
        n180 = Merge Errors(w433, w435) -> (w434:errorcluster)
      }
      frame "Error" {
        # "Error - Check the error message data and respond accordingly. This message is sent by the \"Error Handler\" VIs at the end of each loop in this application."
        n181 = Variant To Data(error in=w480, type=errorcluster {"status"=FALSE, "code"=0, "source"=""} ("error out"), Variant=w479) -> (data=w477:errorcluster, error out=w473:errorcluster)
        n182 = call <vilib>:"Simple Error Handler.vi"("error in (no error)"=w477) -> ()  [unwired: 4 in, 5 out]
        n183 = call-poly "Enqueue Message.vi"("Priority Message? (F)"=TRUE, "Message"="Exit", "Message Queue"=w476) -> ("error out"=w472:errorcluster)  [unwired: 7 in, 1 out]
        n184 = Merge Errors(w472, w473) -> (w471:errorcluster)
      }
      frame "---Copy This Frame---" {
        # "Duplicate this frame when creating new messages.  Change this comment in the duplicated frame to describe this message."
        n185 = Merge Errors(w486) -> (w485:errorcluster)
      }
      frame "Display Setting" {
        # "Duplicate this frame when creating new messages.  Change this comment in the duplicated frame to describe this message."
        n186 = Unbundle By Name(w490) -> ("Hardware Configuration.Sample Rate"=→"Rate (Hz)":dbl, "Hardware Configuration.Max Input"=→"Input (V)":dbl, "Hardware Configuration.Min Input"=→"?":dbl, "Logging Configuration.Author"=→"User":string, "Logging Configuration.Description"=→"Description":string)
        n187 = Merge Errors(w496) -> (w495:errorcluster)
      }
      frame Default {
        # "'Default' case only runs if there is a message that isn't defined in any of the other cases.  Output a programming error."
        n188 = xnode "Error Ring"("parameter 0"=w499) -> ("error out"=w500:errorcluster)
      }
    }
    n189 = call "Error Handler - Message Handling Loop.vi"("error in (no error)"=w237, "Message Queue"=w235) -> ("dup error in"=w236:errorcluster)  [unwired: 8 in, 1 out]
  }
  n190 = while {
    tunnel: w3 -> [w515]
    tunnel: [w511] -> w22
    shift-right: [w514] -> w13
    shift-left: w20 -> [w516]
    stop <- w510 stop-if-true
    # "Event Handling Loop"
    n191 = event shown="[0] \"Settings\": Value Change" {
      selector: w516 -> [_ _ _ _ _ _ _ _ _]
      dyn-events: [_ _ _ _ _ _ _ _ _] -> w514
      timeout: _ -> [_ _ _ _ _ _ _ _ _]
      tunnel: [_ _ _ _ _ _ _ _ TRUE ("Discard?")] -> w510
      tunnel: w515 -> [w518 w522 w527 w531 w534 w537 w541 w547 w548]
      tunnel: [w520 w524 w526 _ w533 w540 _ w542 _] -> w512
      tunnel: [w517 w521 w525 w530 w532 w536 w541 w543 w548] -> w513
      event "Settings": Value Change {
        n192 = event-data() -> ()  [unwired: 1 in, 1 out]
        n193 = call-poly "Enqueue Message.vi"("Message"="Launch Settings Dialog", "Message Queue"=w518) -> ("error out"=w520:errorcluster, "dup Message Queue"=w517:refnum<queue>)  [unwired: 8 in]
      }
      event "Acquire": Value Change {
        n194 = event-data() -> ()  [unwired: 1 in, 1 out]
        n195 = call-poly "Enqueue Message.vi"("Message"="Acquire", "Message Queue"=w522) -> ("error out"=w524:errorcluster, "dup Message Queue"=w521:refnum<queue>)  [unwired: 8 in]
      }
      event "Stop_Acquire": Value Change {
        n196 = event-data() -> ()  [unwired: 1 in, 1 out]
        n197 = call-poly "Enqueue Message.vi"("Message"="Stop_Acquire", "Message Queue"=w527) -> ("error out"=w526:errorcluster, "dup Message Queue"=w525:refnum<queue>)  [unwired: 8 in]
      }
      event "Log": Value Change {
        n198 = event-data() -> ()  [unwired: 1 in, 1 out]
        n199 = call-poly "Enqueue Message.vi"("Message"="Log", "Message Queue"=w531) -> ("dup Message Queue"=w530:refnum<queue>)  [unwired: 8 in, 1 out]
      }
      event "Stop_Log": Value Change {
        n200 = event-data() -> ()  [unwired: 1 in, 1 out]
        n201 = call-poly "Enqueue Message.vi"("Message"="Stop_Log", "Message Queue"=w534) -> ("error out"=w533:errorcluster, "dup Message Queue"=w532:refnum<queue>)  [unwired: 8 in]
      }
      event "Exit": Value Change; Panel Close {
        w538 = TRUE  # Priority Message
        # "The UI Message Loop handles sending the Exit message to other loops."
        n202 = event-data() -> ()  [unwired: 1 in, 1 out]
        n203 = call-poly "Enqueue Message.vi"("Priority Message? (F)"=w538, "Message"="Exit", "Message Queue"=w537) -> ("error out"=w540:errorcluster, "dup Message Queue"=w536:refnum<queue>)  [unwired: 7 in]
      }
      event Application Instance Close {
        n204 = event-data() -> ()  [unwired: 1 in, 1 out]
      }
      event Panel Close? {
        # "Send the 'Confirm Quit' message if the user closes the panel of the VI. Discard the event so the 'Confirm Quit' message has a chance to run."
        n205 = event-data() -> ()  [unwired: 1 in, 1 out]
        n206 = call-poly "Enqueue Message.vi"("Priority Message? (F)"=TRUE, "Message"="Confirm Quit", "Message Queue"=w547) -> ("error out"=w542:errorcluster, "dup Message Queue"=w543:refnum<queue>)  [unwired: 7 in]
        n207 = event-data("Discard?"=TRUE) -> ()  [unwired: 1 in, 1 out]
      }
      event User Event {
        # "The Message Handling Loop processed an \"Exit\" message, which fired this event to stop the Event Handling Loop."
        n208 = event-data() -> ()  [unwired: 1 in, 1 out]
        n209 = local write "Status"("Exit" ("Exit String")) -> ()
      }
    }
    n210 = Wait (ms)(milliseconds to wait=u32 100) -> ()  [unwired: 1 out]
    n211 = call "Error Handler - Event Handling Loop.vi"("error in (no error)"=w512, "Message Queue"=w513) -> ("dup error in"=w511:errorcluster)  [unwired: 8 in, 1 out]
  }
  n212 = call "Acquisition Message Loop.vi"("error in (no error)"=w4, "Data Queue"=w2, "Data Notifier"=w1, "Message Queues"=w16) -> ("error out"=w18:errorcluster)  [unwired: 7 in]
  n213 = call "Logging Message Loop.vi"("error in (no error)"=w4, "Data Queue"=w2, "Message Queues"=w16) -> ("error out"=w15:errorcluster)  [unwired: 8 in]
  n214 = Unregister For Events(event registration refnum=w13, error in=w22) -> (error out=w14:errorcluster)
  n215 = Merge Errors(w14, w23, w18, w15) -> (w21:errorcluster)
  n216 = call "Destroy User Event - Stop.vi"("error in (no error)"=w21, "User Event - Stop"=w19) -> ("error out"=w7:errorcluster)  [unwired: 9 in]
  n217 = disable-structure shown="RUN_TIME_ENGINE==True" {
    disable-tunnel: w7 -> [_ _]
    frame condition #0 {
      # "Call Quit LabVIEW if running as a built application."
      n218 = Quit LabVIEW() -> ()  [unwired: 1 in]
    }
    frame condition #1 (active) {
    }
  }
